vi "Second_min.vi"(8 "error in (no error)":errorcluster, 11 "Array":dbl[](array[numeric])) -> (0 "error IO":errorcluster, 3 "output":dbl)   [LabVIEW 2022 SP3]
uses:
  SI_modules/SI656/SI656.lvclass/SI656.ctl
  39c5035a-b564-434f-9c62-cccc5aca10b8.vi
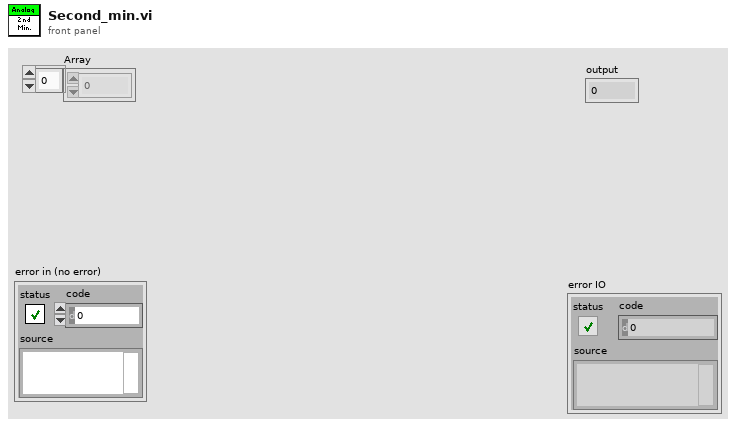
[diagram p1: front panel]
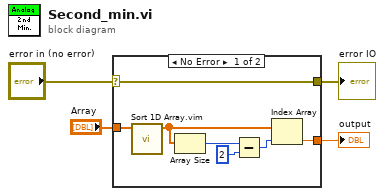
[diagram p0: block diagram]
diagram:
  n1 = case shown="No Error" "error in (no error)" {
    selector: "error in (no error)" -> [w7 w12]
    tunnel: [w7 w12] -> w3
    tunnel: [w6 _] -> w2
    tunnel: "Array" -> [w5 _]
    frame No Error {
      n2 = call "Sort 1D Array.vim"("unsorted array"=w5) -> ("sorted array"=w8:dbl[])  [unwired: 10 in]
      n3 = Array Size(array=w8) -> (size(s)=w9:i32)
      n4 = Subtract(x=w9, y=2) -> (x-y=w11:i32)
      n5 = Index Array(array=w8, index=w11) -> (element=w6:dbl)
    }
    frame Error {
    }
  }
  "error IO" <- w3
  "output" <- w2
